vi "SpatialEventExe.vi"(0 "Devices In":u64[](array[numeric]), 1 "Event Registration Refnum In":refnum<event-registration>, 7 "error in (no error)":errorcluster) -> (16 "Index":i32, 18 "Event?":bool, 19 "phid":u64, 20 "Devices Out":u64[](array[numeric]), 21 "Event Registration Refnum Out":refnum<event-registration>, 23 "Accel Data":dbl[](array[numeric]), 24 "Gyro Data":dbl[](array[numeric]) caption="Angular Rate Data", 25 "Field Str Data":dbl[](array[numeric]) caption="Mag Field Data", 26 "Timestamp":dbl, 27 "error out":errorcluster)   [LabVIEW 2012, in "Phidget Spatial.lvlib"]
doc: "${SpatialData:Header}"
uses:
  <instrlib>/Phidgets/Phidget Spatial/Phidget Spatial.lvlib
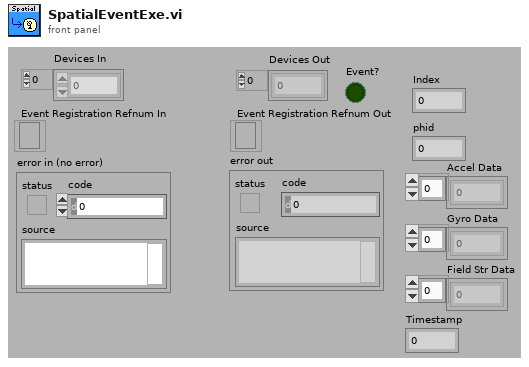
[diagram p1: front panel]
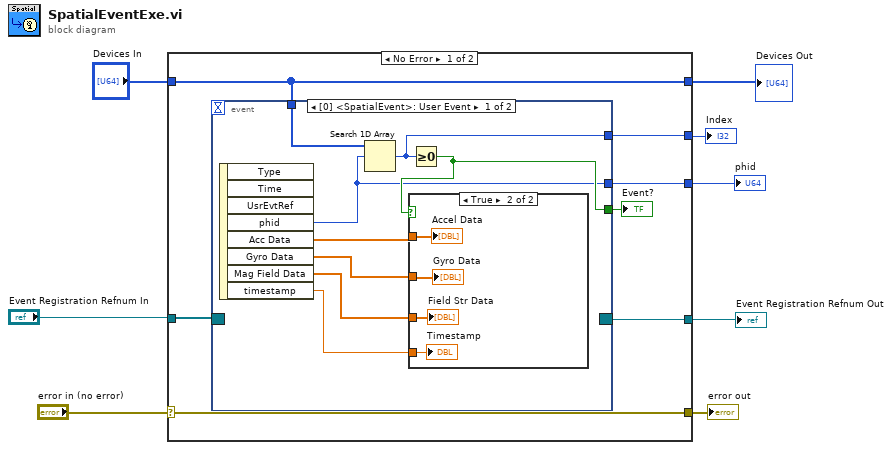
[diagram p0: block diagram]
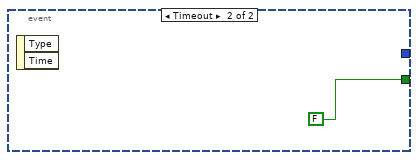
[diagram p3: hidden frame]
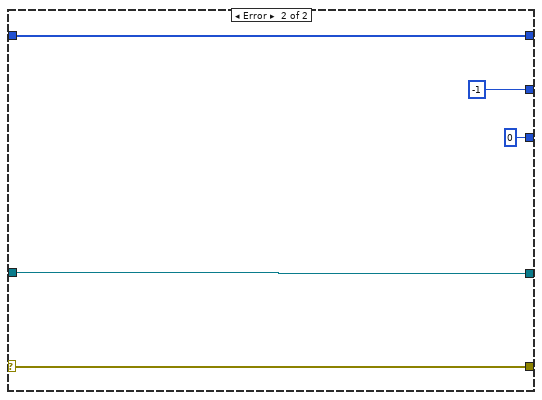
[diagram p4: hidden frame]
diagram:
  n1 = case shown="No Error" "error in (no error)" {
    selector: "error in (no error)" -> [w12 w33]
    tunnel: [w12 w33] -> w7
    tunnel: [w15 w32] -> w1
    tunnel: "Event Registration Refnum In" -> [w14 w32]
    tunnel: [w11 w31] -> w5
    tunnel: "Devices In" -> [w11 w31]
    tunnel: [w10 -1] -> w4
    tunnel: [w9 u64 0 ("phid")] -> w3
    frame No Error {
      n2 = event shown="[0] <SpatialEvent>: User Event" {
        selector: w14 -> [_ _]
        dyn-events: [_ _] -> w15
        timeout: _ -> [_ _]
        tunnel: [w22 FALSE] -> w13
        tunnel: w11 -> [w23 _]
        tunnel: [w21 _] -> w10
        tunnel: [w20 _] -> w9
        event User Event {
          n3 = event-data() -> ("phid"=w20:u64, "Acc Data"=w16:dbl[], "Gyro Data"=w17:dbl[], "Mag Field Data"=w18:dbl[], "timestamp"=w19:dbl)  [unwired: 1 in, 3 out]
          n4 = Search 1D Array(1D array=w23, element=w20) -> (index of element=w21:i32)  [unwired: 1 in]
          n5 = Greater Or Equal To 0?(x=w21) -> (x >= 0?=w22:bool)
          n6 = case shown="True" w22 {
            tunnel: w16 -> [_ w27]
            tunnel: w19 -> [_ w24]
            tunnel: w17 -> [_ w26]
            tunnel: w18 -> [_ w25]
            frame False {
            }
            frame True {
              "Accel Data" <- w27
              "Gyro Data" <- w26
              "Field Str Data" <- w25
              "Timestamp" <- w24
            }
          }
        }
        event Timeout {
          n7 = event-data() -> ()  [unwired: 1 in, 2 out]
        }
      }
      "Event?" <- w13
    }
    frame Error {
    }
  }
  "error out" <- w7
  "Devices Out" <- w5
  "Index" <- w4
  "phid" <- w3
  "Event Registration Refnum Out" <- w1
